vi "lab8.vi"() -> ()   [LabVIEW 2016]
panel:
  out "ang 2":dynamicdata(graph)
  out "photo2":dynamicdata(graph)
  out "Piezer 2":dynamicdata(graph)
  out "Waveform Graph 2":dynamicdata(graph)
  out "Waveform Graph":dynamicdata(graph)
  out "photot1 2":dbl
  out "Piezer":dynamicdata(graph)
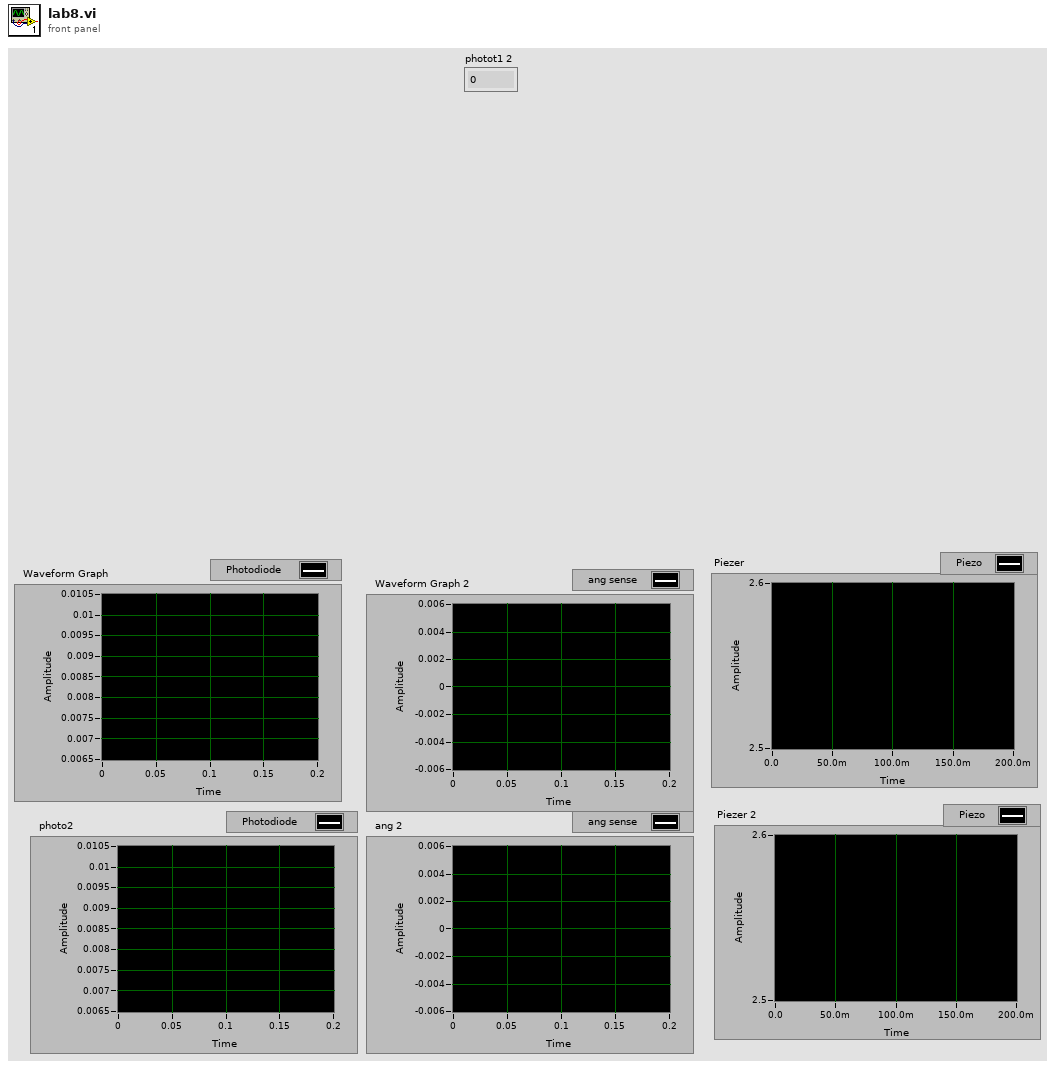
[diagram p1: front panel]
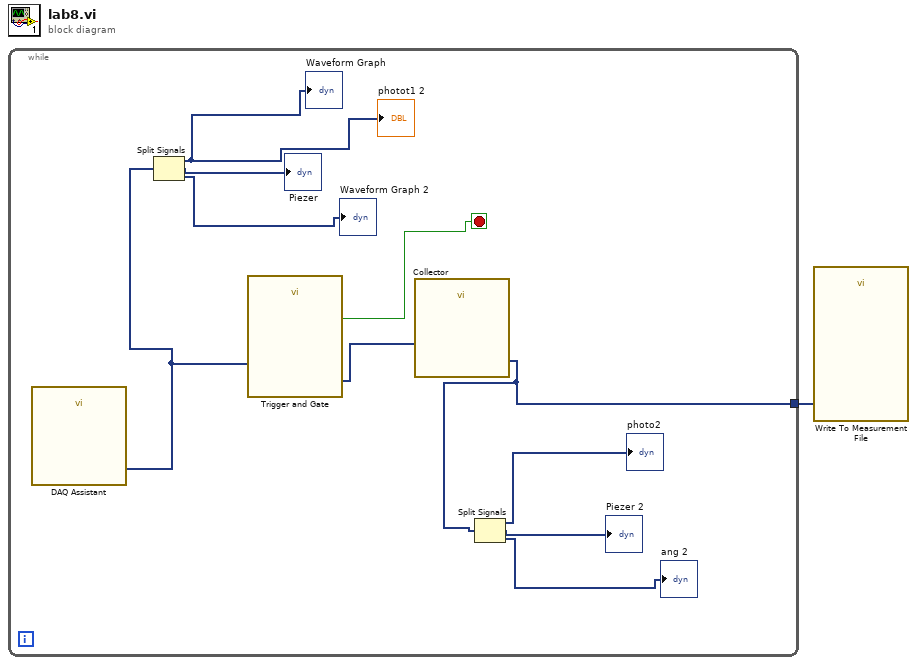
[diagram p0: block diagram]
diagram:
  n1 = while {
    tunnel: [w2] -> w1
    stop <- w8 stop-if-true
    n2 = call "DAQ Assistant"() -> ("data"=w11:dynamicdata)  [unwired: 17 in, 2 out]
    n3 = Split Signals(w11) -> (→"photot1 2" →"Waveform Graph":dynamicdata, →"Piezer":dynamicdata, →"Waveform Graph 2":dynamicdata)  [unwired: 3 in]
    n4 = call "Trigger and Gate"("Signals"=w11) -> ("Triggered Signals"=w10:dynamicdata, "Data Available"=w8:bool)  [unwired: 7 in, 2 out]
    n5 = call "Collector"("Signals"=w10) -> ("Collected Signals"=w2:dynamicdata)  [unwired: 9 in, 1 out]
    n6 = Split Signals(w2) -> (→"photo2":dynamicdata, →"Piezer 2":dynamicdata, →"ang 2":dynamicdata)  [unwired: 3 in]
  }
  n7 = call "Write To Measurement File"("Signals"=w1) -> ()  [unwired: 16 in, 3 out]
